vi "Example OpenCV Object Tracking2.0.vi"() -> ()   [LabVIEW 2014]
uses:
  vi.lib/Q-WaveSystems/QwaveSys Raspberry Pi for LabVIEW Home-Education/QwaveSys Raspberry Pi Library.lvlib
panel:
  out "found":u32[][](array[numeric])
  in  "webcamnum":i32
  in  "Color  Upper":u32(colorbox)=7001344
  in  "Color  Lower":u32(colorbox)=16777088
  out "Output":picture
  in  "Blank Button":bool
  out "2D Picture":picture
  # "X"
  # "Y"
  # "R"
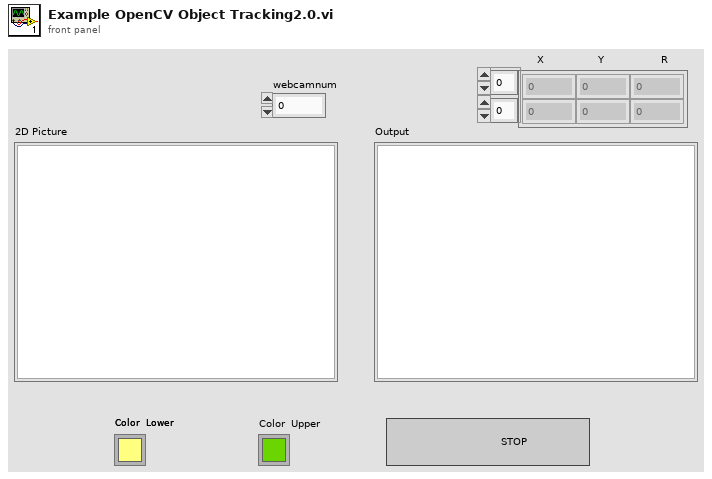
[diagram p1: front panel]
types:
  T1 = typedef "imagedata.ctl" = cluster{"image type":i32, "image depth":i32, "image":u8[], "mask":u8[], "colors":u32[], "Rectangle":cluster{"left":i16, "top":i16, "right":i16, "bottom":i16}}
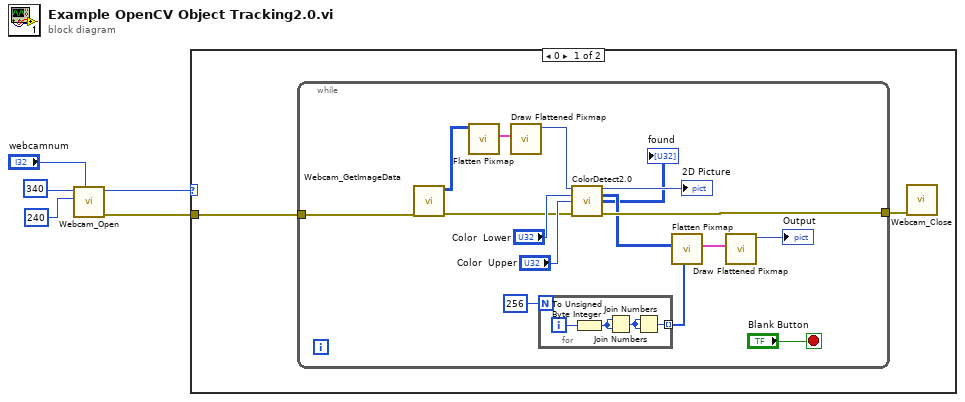
[diagram p0: block diagram]
diagram:
  n1 = call "Webcam_Open.vi"("webcamnum"="webcamnum", "height"=u32 240, "width"=u32 340) -> ("error out"=w3:errorcluster, "return type"=w2:i32)  [unwired: 7 in]
  n2 = case shown="0" w2 {
    tunnel: w3 -> [w6 _]
    frame 0 {
      n3 = while {
        tunnel: [w22] -> w7
        tunnel: w6 -> [w21]
        stop <- "Blank Button" stop-if-true
        n4 = call "Webcam_GetImageData.vi"("error in (no error)"=w21) -> ("error out"=w10:errorcluster, "image24bits"=w9:u32[][])  [unwired: 8 in, 1 out]
        n5 = call <vilib>:"Flatten Pixmap.vi"("24-bit pixmap"=w9) -> ("image data"=w20:T1)  [unwired: 10 in]
        n6 = call <vilib>:"Draw Flattened Pixmap.vi"("image data"=w20) -> ("new picture"=w16:picture)  [unwired: 8 in]
        n7 = for {
          N: 256 -> [_]
          tunnel: [w27] -> w11 mode=indexing
          i -> [w25]
          n8 = To Unsigned Byte Integer(number=w25) -> (unsigned 8bit integer=w24:u8)
          n9 = Join Numbers(hi=w24, lo=w24) -> ((hi.lo)=w26:u16)
          n10 = Join Numbers(hi=w26, lo=w26) -> ((hi.lo)=w27:u32)
        }
        n11 = call "ColorDetect2.0.vi"("new picture"=w16, "Color 1 Lower"="Color  Lower", "Color 1 Upper"="Color  Upper", "error in (no error)"=w10) -> ("out picture"=→"2D Picture":picture, "image"=w12:u8[][], "found"=→"found":u32[][], "error out"=w22:errorcluster)  [unwired: 8 in]
        n12 = call <vilib>:"Flatten Pixmap.vi"("colors"=w11, "8-bit pixmap"=w12) -> ("image data"=w19:T1)  [unwired: 9 in]
        n13 = call <vilib>:"Draw Flattened Pixmap.vi"("image data"=w19) -> ("new picture"=→"Output":picture)  [unwired: 8 in]
      }
      n14 = call "Webcam_Close.vi"("error in (no error)"=w7) -> ()  [unwired: 10 in, 1 out]
    }
    frame -1, Default {
      # "No Camera Found"
    }
  }
